vi "Configure VM Trigger.vi"(5 "External Trigger Polarity (0: Positive)":i32(ring) items=["Positive", "Negative"], 6 "External Trigger Delay (0 s)":dbl, 7 "External Trigger Source (0: EPTrigger1)":i32(ring) items=["EPTrigger1", "EPTrigger2"], 8 "error in (no error)":errorcluster, 9 "Trigger Type (0: Free)":i32(ring) items=["Free", "Trigger"], 10 "Trigger Source (2: External)":i32(ring)=2 items=["Key", "Bus", "External"], 11 "VISA resource name":refnum<visa-resource-name>) -> (0 "error out":errorcluster, 3 "VISA resource name out":refnum<visa-resource-name>)   [LabVIEW 2014, in "Agilent PSG MXG Series.lvlib"]
doc: "Configure output trigger settings.\n\n<B>Notes:</B>\n(1) This VI is valid only in N5172B and N5182B that install <B>Option 660</B>."
uses:
  Agilent PSG MXG Series.lvlib
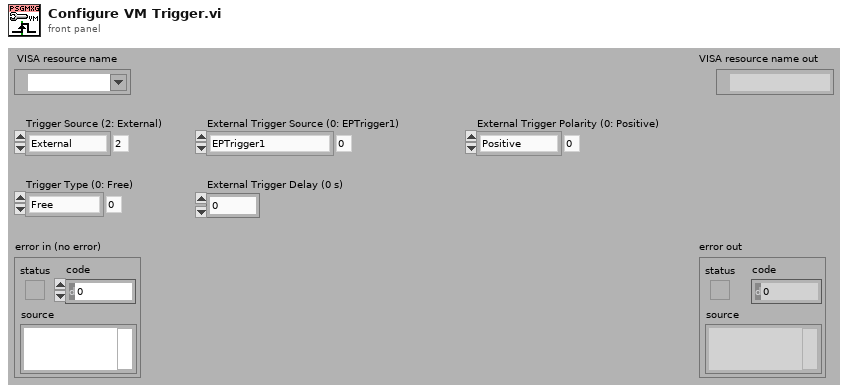
[diagram p1: front panel]
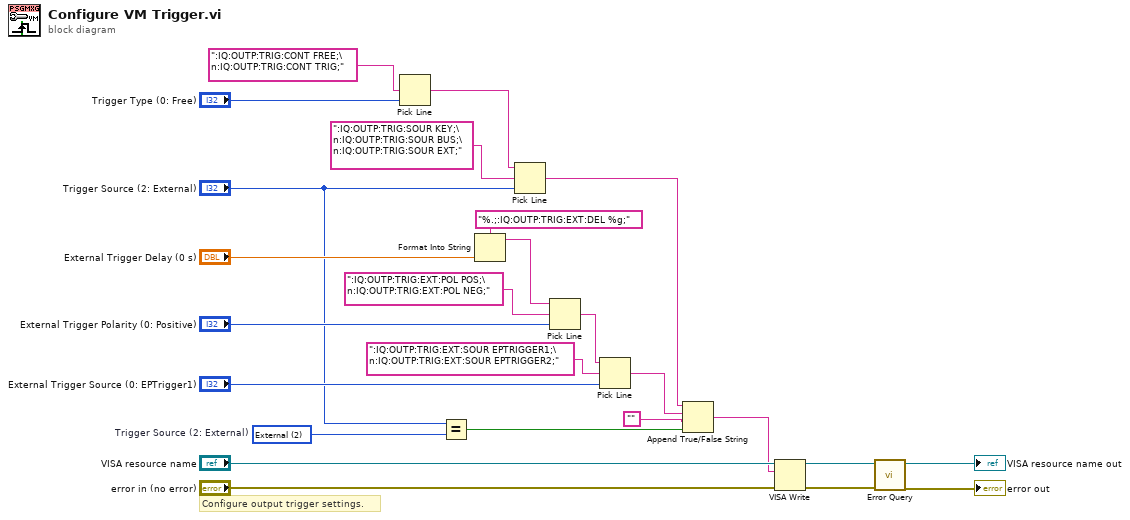
[diagram p0: block diagram]
diagram:
  w7 = 2 items=["Key", "Bus", "External"]  # Trigger Source (2: External)
  # "Configure output trigger settings."
  n1 = Pick Line(multi-line string=":IQ:OUTP:TRIG:CONT FREE;\n:IQ:OUTP:TRIG:CONT TRIG;", line index="Trigger Type (0: Free)") -> (output string=w9:string)  [unwired: 1 out]
  n2 = Equal?(x="Trigger Source (2: External)", y=w7) -> (x = y?=w5:bool)
  n3 = Format Into String(format string="%.;:IQ:OUTP:TRIG:EXT:DEL %g;", "External Trigger Delay (0 s)") -> (resulting string=w19:string)  [unwired: 2 in, 1 out]
  n4 = Pick Line(string ("")=w9, multi-line string=":IQ:OUTP:TRIG:SOUR KEY;\n:IQ:OUTP:TRIG:SOUR BUS;\n:IQ:OUTP:TRIG:SOUR EXT;", line index="Trigger Source (2: External)") -> (output string=w3:string)
  n5 = Pick Line(string ("")=w19, multi-line string=":IQ:OUTP:TRIG:EXT:POL POS;\n:IQ:OUTP:TRIG:EXT:POL NEG;", line index="External Trigger Polarity (0: Positive)") -> (output string=w8:string)
  n6 = Pick Line(string ("")=w8, multi-line string=":IQ:OUTP:TRIG:EXT:SOUR EPTRIGGER1;\n:IQ:OUTP:TRIG:EXT:SOUR EPTRIGGER2;", line index="External Trigger Source (0: EPTrigger1)") -> (output string=w4:string)
  n7 = Append True/False String(1:w5, 2:"", 3:w4, 4:w3) -> (0:w1:string)
  n8 = VISA Write(VISA resource name="VISA resource name", write buffer=w1, error in (no error)="error in (no error)") -> (VISA resource name out=w15:refnum<visa-resource-name>, error out=w14:errorcluster)  [unwired: 1 out]
  n9 = call "Error Query.vi"("error in (no error)"=w14, "VISA resource name"=w15) -> ("error out"=→"error out":errorcluster, "VISA resource name out"=→"VISA resource name out":refnum<visa-resource-name>)  [unwired: 8 out]
